vi "Print VI to Html and Display.vi"(8 "错误输入（无错误）":errorcluster, 9 "选择":T1={"添加？"=FALSE, "格式"=enum."Custom", "图像格式"=enum."PNG", "图像深度"=8, "浏览器显示"=FALSE} {"图像深度" items=["1位、黑白"=1, "4位、16色"=4, "8位、256色"=8, "24位、真彩色"=24]}, 10 "HTML文件路径":path, 11 "VI Ref":refnum<vi>) -> (0 "错误输出":errorcluster)   [LabVIEW 2012, in "VIRef.lvlib"]
uses:
  VIRef.lvlib
  <vilib>/Platform/browser.llb/Open URL in Default Browser (path).vi
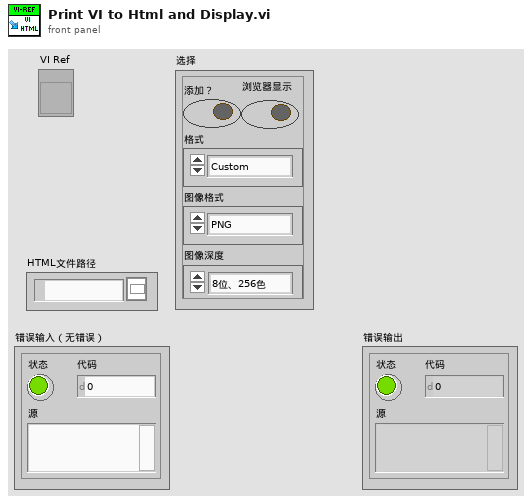
[diagram p1: front panel]
types:
  T1 = cluster{"添加？":bool, "格式":enum32{"Custom", "Standard", "Using Panel", "Using SubVI", "Complete"}, "图像格式":enum32{"PNG", "JPEG", "GIF"}, "图像深度":i32, "浏览器显示":bool}
  T2 = enum32{"Custom", "Standard", "Using Panel", "Using SubVI", "Complete"}
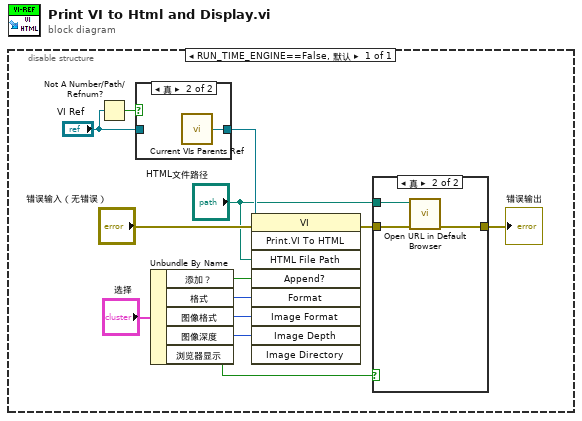
[diagram p0: block diagram]
diagram:
  n1 = disable-structure shown="RUN_TIME_ENGINE==False, 默认" {
    frame condition #0 (active) {
      n2 = Not A Number/Path/Refnum?(number/path/refnum="VI Ref") -> (NaN/Path/Refnum?=w13:bool)
      n3 = case shown="真" w13 {
        tunnel: [w18 w19] -> w5
        tunnel: "VI Ref" -> [w18 _]
        frame False {
        }
        frame True {
          n4 = call "Current VIs Parents Ref.vi"() -> ("Calling VI's Reference"=w19:refnum<vi>)  [unwired: 2 in]
        }
      }
      n5 = Unbundle By Name("选择") -> ("添加？"=w10:bool, "格式"=w9:T2, "图像格式"=w8:enum32{"PNG", "JPEG", "GIF"}, "图像深度"=w7:i32, "浏览器显示"=w6:bool)
      n6 = invoke class="VI" method="Print.VI To HTML"(reference=w5, error in="错误输入（无错误）", "HTML File Path"="HTML文件路径", "Append?"=w10, "Format"=w9, "Image Format"=w8, "Image Depth"=w7) -> (error out=w3:errorcluster)  [unwired: 2 in, 8 out]
      n7 = case shown="真" w6 {
        tunnel: "HTML文件路径" -> [_ w17]
        tunnel: w3 -> [w14 w16]
        tunnel: [w14 w15] -> w2
        frame False {
        }
        frame True {
          n8 = call-poly <vilib>:"Open URL in Default Browser.vi"("error in (no error)"=w16, "path"=w17) -> ("error out"=w15:errorcluster)  [unwired: 4 in, 1 out]
        }
      }
      "错误输出" <- w2
    }
  }
